vi "s-box.vi"(0 "red in":dbl[](array[numeric]), 1 "green in":dbl[](array[numeric]), 2 "blue in":dbl[](array[numeric]), 3 "x":dbl[](array[numeric]), 4 "y":dbl[](array[numeric]), 5 "z":dbl[](array[numeric]), 6 "Numeric":i32) -> (17 "red out":i32[](array[numeric]), 18 "green out":i32[](array[numeric]), 19 "blue out":i32[](array[numeric]))   [LabVIEW 2019]
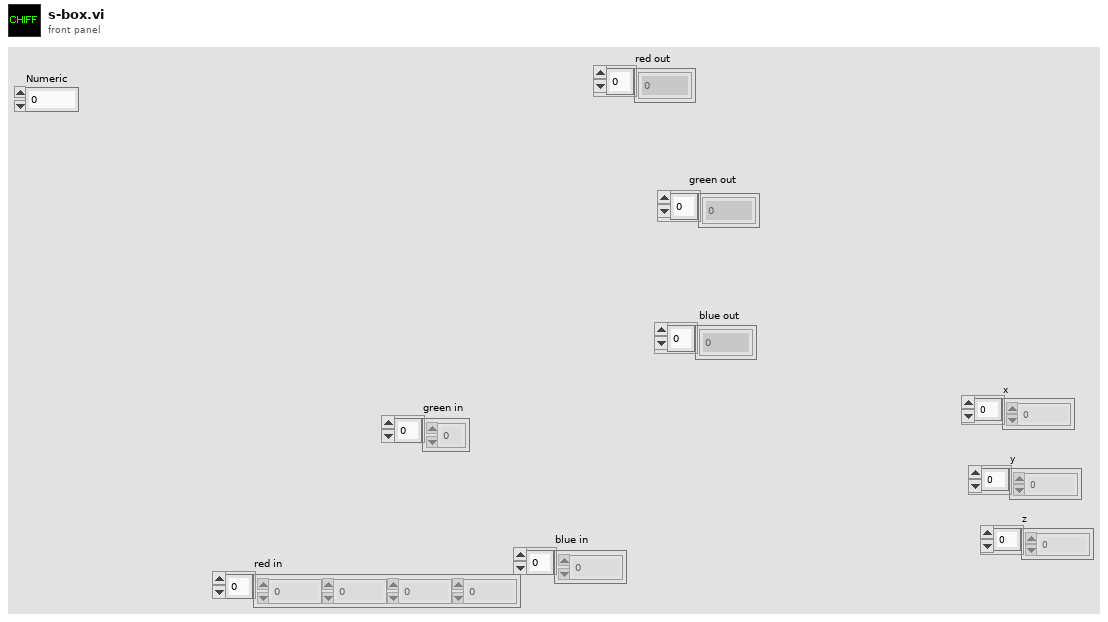
[diagram p1: front panel]
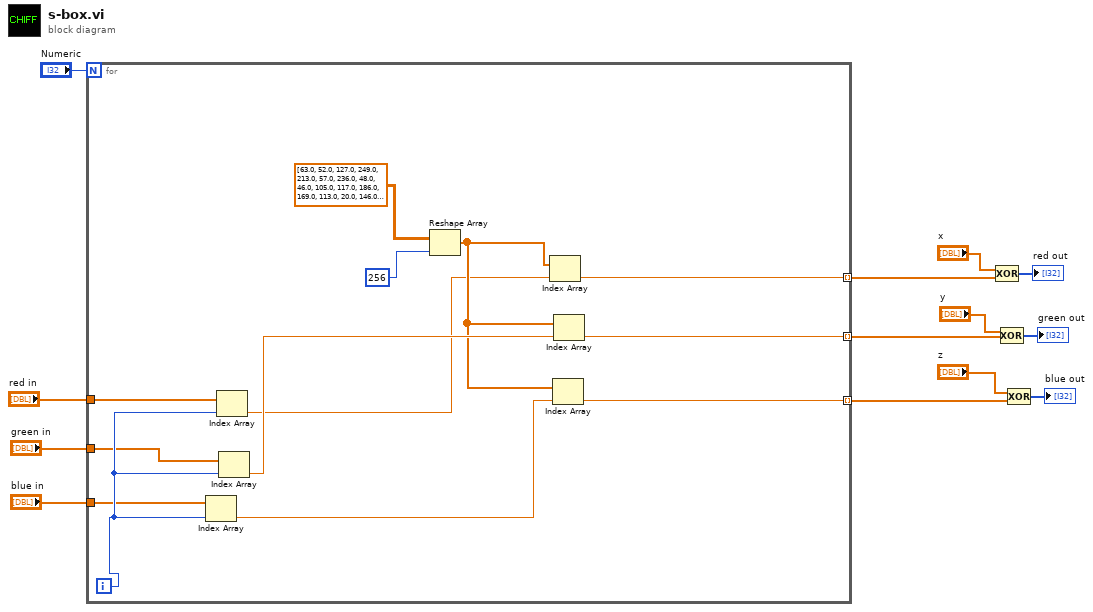
[diagram p0: block diagram]
diagram:
  n1 = for {
    N: "Numeric" -> [_]
    tunnel: "red in" -> [w20]
    tunnel: "green in" -> [w19]
    tunnel: "blue in" -> [w18]
    tunnel: [w16] -> w9 mode=indexing
    tunnel: [w15] -> w5 mode=indexing
    tunnel: [w14] -> w4 mode=indexing
    i -> [w21]
    n2 = Index Array(array=w18, index=w21) -> (element=w17:dbl)
    n3 = Index Array(array=w20, index=w21) -> (element=w23:dbl)
    n4 = Index Array(array=w19, index=w21) -> (element=w26:dbl)
    n5 = Reshape Array(dbl[][] [[63.0, 52.0, 127.0, 249.0, 213.0, 57.0, 236.0, 48.0, 46.0, 105.0, 117.0, 186.0, 169.0, 113.0, 20.0, 146.0], [224.0, 42.0, 83.0, 49.0, 33.0, 137.0, 8.0, 37.0, 208.0, 97.0, 69.0, 247.0, 88.0, 13.0, 73.0, 84.0], [75.0, 158.0, 217.0, 16.0, 136.0, 243.0, 214.0, 176.0, 139.0, 0.0, 96.0, 32.0, 98.0, 68.0, 163.0, 51.0], [120.0, 228.0, 156.0, 138.0, 44.0, 9.0, 235.0, 191.0, 115.0, 161.0, 221.0, 14.0, 193.0, 147.0, 40.0, 11.0], [167.0, 35.0, 123.0, 19.0, 34.0, 78.0, 86.0, 76.0, 184.0, 17.0, 95.0, 153.0, 143.0, 155.0, 178.0, 54.0], [227.0, 27.0, 230.0, 112.0, 216.0, 134.0, 248.0, 200.0, 65.0, 125.0, 30.0, 58.0, 199.0, 1.0, 244.0, 103.0], [47.0, 238.0, 203.0, 5.0, 108.0, 10.0, 232.0, 36.0, 85.0, 149.0, 222.0, 25.0, 255.0, 162.0, 180.0, 70.0], [121.0, 177.0, 104.0, 196.0, 187.0, 64.0, 166.0, 56.0, 145.0, 28.0, 174.0, 171.0, 79.0, 189.0, 114.0, 124.0], [234.0, 66.0, 12.0, 205.0, 126.0, 245.0, 22.0, 183.0, 210.0, 106.0, 170.0, 18.0, 250.0, 182.0, 119.0, 190.0], [77.0, 72.0, 194.0, 130.0, 168.0, 89.0, 185.0, 173.0, 172.0, 82.0, 150.0, 43.0, 142.0, 231.0, 99.0, 144.0], [165.0, 135.0, 118.0, 206.0, 220.0, 23.0, 80.0, 204.0, 62.0, 53.0, 229.0, 225.0, 2.0, 151.0, 116.0, 159.0], [61.0, 55.0, 179.0, 100.0, 246.0, 71.0, 253.0, 198.0, 202.0, 188.0, 15.0, 133.0, 81.0, 24.0, 109.0, 39.0], [110.0, 212.0, 92.0, 128.0, 181.0, 233.0, 129.0, 239.0, 209.0, 4.0, 90.0, 107.0, 251.0, 3.0, 7.0, 41.0], [218.0, 197.0, 215.0, 237.0, 94.0, 254.0, 67.0, 207.0, 192.0, 91.0, 164.0, 157.0, 141.0, 87.0, 122.0, 131.0], [242.0, 211.0, 26.0, 223.0, 140.0, 111.0, 201.0, 241.0, 132.0, 160.0, 219.0, 59.0, 29.0, 45.0, 240.0, 101.0], [226.0, 148.0, 175.0, 50.0, 152.0, 6.0, 60.0, 102.0, 195.0, 74.0, 31.0, 38.0, 21.0, 252.0, 93.0, 154.0]], 256 ("dimension size")) -> (w24:dbl[])
    n6 = Index Array(array=w24, index=w23) -> (element=w16:dbl)
    n7 = Index Array(array=w24, index=w17) -> (element=w14:dbl)
    n8 = Index Array(array=w24, index=w26) -> (element=w15:dbl)
  }
  n9 = Compound Arithmetic op=XOR("x", w9) -> (→"red out":i32[])
  n10 = Compound Arithmetic op=XOR("y", w5) -> (→"green out":i32[])
  n11 = Compound Arithmetic op=XOR("z", w4) -> (→"blue out":i32[])
